vi "Post VI Refnum.vi"(8 "error in (no error)":errorcluster, 10 "VI Refnum":refnum<vi>, 11 "Analyser in":refnum<class "Analyser.lvclass">) -> (0 "error out":errorcluster, 3 "Analyser out":refnum<class "Analyser.lvclass">)   [LabVIEW 2020, in "Analyser.lvlib" / "Analyser.lvclass"]
uses:
  Analyser.lvclass
  C:/Program Files/National Instruments/LabVIEW 2020/vi.lib/ActorFramework/Actor/Actor.lvclass
  <vilib>/ActorFramework/Actor/Actor.lvclass/Actor.ctl
  Interface/DeviceDock Messages/InsertDevicePanel Msg/InsertDevicePanel Msg.lvclass/InsertDevicePanel Msg.ctl
  <vilib>/ActorFramework/Message Enqueuer/Message Enqueuer.lvclass/Message Enqueuer.ctl
  <vilib>/ActorFramework/Message Enqueuer/Enqueue.vi
  Interface/DeviceDock Messages/InsertDevicePanel Msg/InsertDevicePanel Msg.lvclass
  C:/Program Files/National Instruments/LabVIEW 2020/vi.lib/ActorFramework/Message/Message.lvclass
  <vilib>/ActorFramework/Message Priority Queue/Priority Enqueue.vi
  <vilib>/ActorFramework/Actor/Actor.lvclass
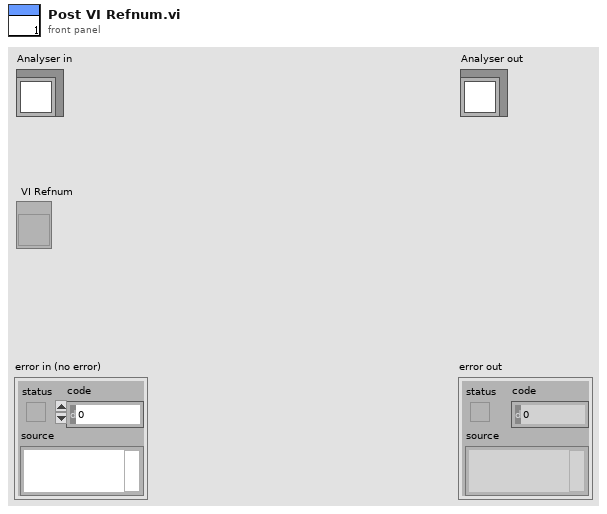
[diagram p1: front panel]
types:
  T1 = enum32{"Invalid", "Standard", "Closed", "Hidden", "Minimized", "Maximized"}
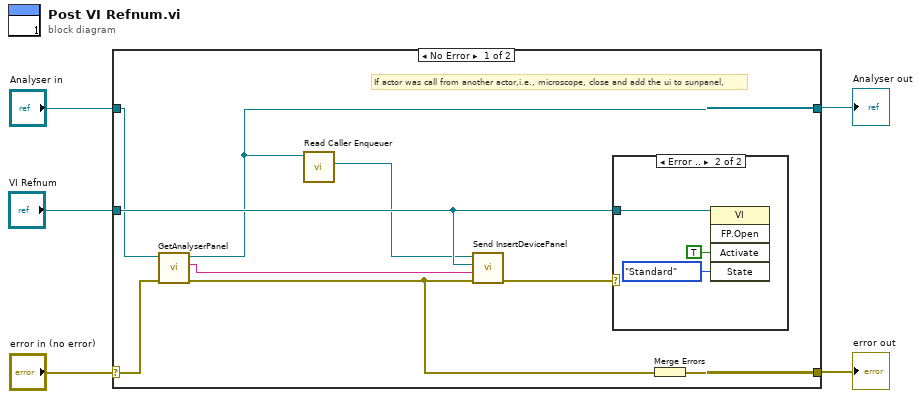
[diagram p0: block diagram]
diagram:
  n1 = case shown="No Error" "error in (no error)" {
    selector: "error in (no error)" -> [w12 w19]
    tunnel: [w14 w19] -> w4
    tunnel: [w8 w18] -> w5
    tunnel: "Analyser in" -> [w7 w18]
    tunnel: "VI Refnum" -> [w13 _]
    frame No Error {
      # "If actor was call from another actor,i.e., microscope, close and add the ui to sunpanel,"
      n2 = call-dynamic "GetAnalyserPanel.vi"("error in (no error)"=w12, "Analyser in"=w7) -> ("error out"=w9:errorcluster, "Panel"=w6:string, "Analyser out"=w8:refnum<class "Analyser.lvclass">)  [unwired: 7 in]
      n3 = call <vilib>:"Read Caller Enqueuer.vi"("Actor"=w8) -> ("Caller Enqueuer"=w11:refnum<class "Message Enqueuer.lvclass">)  [unwired: 10 in]
      n4 = call "Send InsertDevicePanel.vi"("error in (no error)"=w9, "Panel"=w6, "VI Refnum"=w13, "Message Enqueuer"=w11) -> ("error out"=w10:errorcluster)  [unwired: 6 in, 1 out]
      n5 = case shown="Error .." w10 {
        tunnel: w13 -> [_ w17]
        frame No Error {
        }
        frame Error {
          n6 = invoke class="VI" method="FP.Open"(reference=w17, "Activate"=TRUE ("Activate?"), "State"=T1."Standard") -> ()  [unwired: 2 in, 5 out]
        }
      }
      n7 = Merge Errors(w9) -> (w14:errorcluster)
    }
    frame Error {
    }
  }
  "error out" <- w4
  "Analyser out" <- w5
